vi "Parse input.vi"(11 "Input":string) -> (2 "Distances":u64[](array[numeric]), 3 "Times":u64[](array[numeric]))   [LabVIEW 2021]
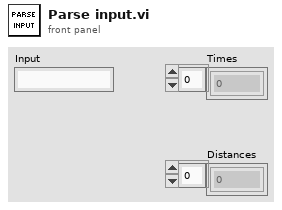
[diagram p1: front panel]
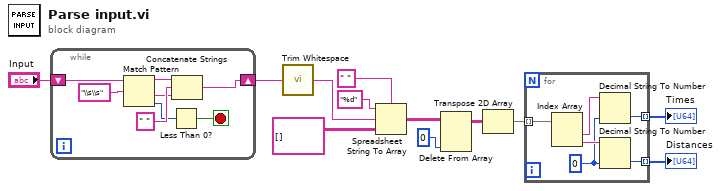
[diagram p0: block diagram]
diagram:
  n1 = while {
    shift-right: [w15] -> w4
    shift-left: "Input" -> [w20]
    stop <- w13 stop-if-true
    n2 = Match Pattern(string=w20, regular expression="\\s\\s") -> (before substring=w18:string, after substring=w16:string, offset past match=w14:i32)  [unwired: 1 in, 1 out]
    n3 = Less Than 0?(x=w14) -> (x < 0?=w13:bool)
    n4 = Concatenate Strings(w18, " " ("delimiter (Tab)"), w16) -> (w15:string)
  }
  n5 = call <vilib>:"Trim Whitespace.vi"("string"=w4) -> ("trimmed string"=w12:string)  [unwired: 1 in]
  n6 = Spreadsheet String To Array(delimiter (Tab)=" ", format string="%d", spreadsheet string=w12, array type (2D Dbl)=string[][] []) -> (array=w6:string[][])
  n7 = Delete From Array(array=w6, index (col)=0 ("disabled index (col)")) -> (array with subset deleted=w8:string[][])  [unwired: 2 in, 1 out]
  n8 = Transpose 2D Array(2D array=w8) -> (transposed array=w11:string[][])
  n9 = for {
    tunnel: w11 -> [w26] mode=indexing
    tunnel: [w23] -> w10 mode=indexing
    tunnel: [w22] -> w9 mode=indexing
    w21 = u64 0 ("default (0 I32)")
    n10 = Index Array(array=w26) -> (element #1=w25:string, element #2=w24:string)  [unwired: 2 in]
    n11 = Decimal String To Number(string=w25, default (0L)=w21) -> (number=w22:u64)  [unwired: 1 in, 1 out]
    n12 = Decimal String To Number(string=w24, default (0L)=w21) -> (number=w23:u64)  [unwired: 1 in, 1 out]
  }
  "Distances" <- w10
  "Times" <- w9
